vi "Channel2TraceNr.vi"(9 "channel names":string[](array[string])) -> (1 "Unique trace numbers":dbl[](array[numeric]))   [LabVIEW 2018]
uses:
  <vilib>/Analysis/polynomials.llb/Unique Numbers and Multiplicity (DBL).vi
  <vilib>/regexp/Match Regular Expression.xnode
  <vilib>/Analysis/NI_AALPro.lvlib
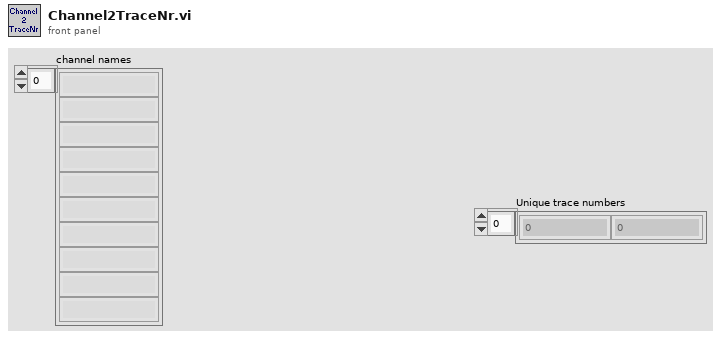
[diagram p1: front panel]
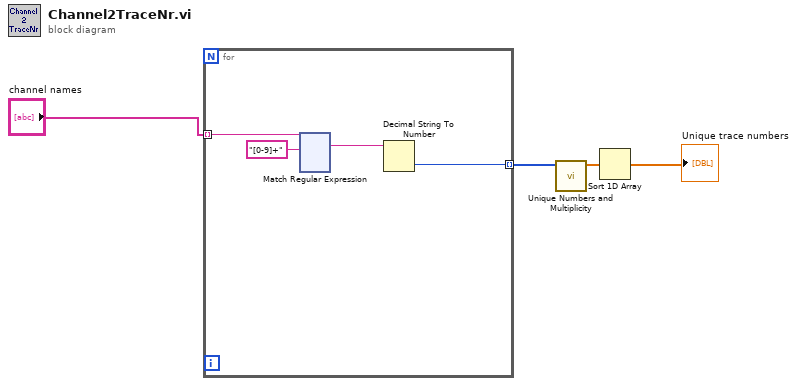
[diagram p0: block diagram]
diagram:
  n1 = for {
    tunnel: "channel names" -> [w8] mode=indexing
    tunnel: [w7] -> w4 mode=indexing
    n2 = xnode "Match Regular Expression"("input string"=w8, "regular expression"="[0-9]+") -> ("whole match"=w5:string)  [unwired: 4 in, 4 out]
    n3 = Decimal String To Number(string=w5) -> (number=w7:i32)  [unwired: 2 in, 1 out]
  }
  n4 = call-poly <vilib>:"Unique Numbers and Multiplicity.vi"("Numbers"=w4) -> ("Unique Numbers"=w3:dbl[])  [unwired: 8 in, 2 out]
  n5 = Sort 1D Array(array=w3) -> (sorted array=→"Unique trace numbers":dbl[])
